vi "projectile_motion_MathScript_ver0.vi"() -> ()   [LabVIEW 2011]
uses:
  <vilib>/imath/engines/lvmath/Plug In/_Char/NIMS_CH_character datatype.ctl
  Instance           1 43Saved   Worked Example--Function Generation .vi
  <vilib>/Utility/file.llb/Write To Spreadsheet File (DBL).vi
  <vilib>/imath/engines/lvmath2/RunTimeEngine/ErrorHandling/NIMS_Finalize Error.vi
  <vilib>/imath/engines/lvmath2/RunTimeEngine/Managers/WorkSpace/UID Generator.vi
  <vilib>/imath/engines/lvmath2/RunTimeEngine/CommandStatement/NIMS_CommandStatement_MaskErr.vi
  <vilib>/imath/engines/lvmath2/RunTimeEngine/Managers/SymbolTable/Clear UID.vi
  <vilib>/imath/engines/lvmath2/RunTimeEngine/NodeEndStatement/NIMS_NodeEndStatement_Output.vi
  <instcachedir>/0/NIMS_NodeEndStatement_Output_53EC0D466D134D7ABD903AC30B43404B.lvgen/NIMS_NodeEndStatement_Output_53EC0D466D134D7ABD903AC30B43404B_001.vi
  <instcachedir>/0/NIMS_NodeEndStatement_Output_53EC0D466D134D7ABD903AC30B43404B.lvgen/NIMS_NodeEndStatement_Output_53EC0D466D134D7ABD903AC30B43404B_005.vi
  <vilib>/imath/engines/lvmath2/RunTimeEngine/ReplaceToken/NIMS_Replace - Check Linear.vi
  <instcachedir>/0/NIMS_Replace - Check Linear_276AD648BD064726893CCF9ED6E2A728.lvgen/NIMS_Replace - Check Linear_276AD648BD064726893CCF9ED6E2A728_006.vi
  <vilib>/imath/engines/lvmath2/RunTimeEngine/ReplaceToken/NIMS_Replace - Size Check _(_)=S.vi
  <instcachedir>/0/NIMS_Replace - Size Check _(_)=S_9ABE7AF2D26C43EAA05192D5C1E6C624.lvgen/NIMS_Replace - Size Check _(_)=S_9ABE7AF2D26C43EAA05192D5C1E6C624_004.vi
  <vilib>/imath/engines/lvmath2/RunTimeEngine/ReplaceToken/NIMS_Replace - V(S)=S.vi
  <instcachedir>/0/NIMS_Replace - V(S)=S_16B13A4565AB46F59881314645612498.lvgen/NIMS_Replace - V(S)=S_16B13A4565AB46F59881314645612498_002.vi
  <vilib>/imathl/engines/lvmath/Functions/Error Handling/Create Error.vi
  <instcachedir>/0/NIMS_Replace - Check Linear_276AD648BD064726893CCF9ED6E2A728.lvgen/NIMS_Replace - Check Linear_276AD648BD064726893CCF9ED6E2A728_001.vi
  <instcachedir>/0/NIMS_Replace - Size Check _(_)=S_9ABE7AF2D26C43EAA05192D5C1E6C624.lvgen/NIMS_Replace - Size Check _(_)=S_9ABE7AF2D26C43EAA05192D5C1E6C624_000.vi
  <instcachedir>/0/NIMS_Replace - V(S)=S_16B13A4565AB46F59881314645612498.lvgen/NIMS_Replace - V(S)=S_16B13A4565AB46F59881314645612498_000.vi
  <vilib>/imath/engines/lvmath2/RunTimeEngine/VariableToken/Read/NIMS_Get Elements - RV(_) - Check.vi
  <instcachedir>/0/NIMS_Get Elements - RV(_) - Check_B511B9D8E05044FE80F9F088FE24B20C.lvgen/NIMS_Get Elements - RV(_) - Check_B511B9D8E05044FE80F9F088FE24B20C_003.vi
  <vilib>/imath/engines/lvmath2/RunTimeEngine/CommandStatement/MC_CommandStatement_break.vi
  <instcachedir>/0/NIMS_Replace - Check Linear_276AD648BD064726893CCF9ED6E2A728.lvgen/NIMS_Replace - Check Linear_276AD648BD064726893CCF9ED6E2A728_002.vi
  <vilib>/imath/engines/lvmath2/RunTimeEngine/ArithmeticOperatorToken/NIMS_ArithmeticOperator_power(S).vi
  <instcachedir>/0/NIMS_ArithmeticOperator_power(S)_92C23AD9D71943099E05992575E16482.lvgen/NIMS_ArithmeticOperator_power(S)_92C23AD9D71943099E05992575E16482_010.vi
  <instcachedir>/0/NIMS_Replace - Size Check _(_)=S_9ABE7AF2D26C43EAA05192D5C1E6C624.lvgen/NIMS_Replace - Size Check _(_)=S_9ABE7AF2D26C43EAA05192D5C1E6C624_001.vi
  <instcachedir>/0/NIMS_Replace - V(S)=S_16B13A4565AB46F59881314645612498.lvgen/NIMS_Replace - V(S)=S_16B13A4565AB46F59881314645612498_001.vi
  <vilib>/imath/engines/lvmath2/RunTimeEngine/ErrorHandling/NIMS_Create Error From Enums.vi
  <instcachedir>/0/NIMS_Get Elements - RV(_) - Check_B511B9D8E05044FE80F9F088FE24B20C.lvgen/NIMS_Get Elements - RV(_) - Check_B511B9D8E05044FE80F9F088FE24B20C_000.vi
  <vilib>/imath/engines/lvmath2/RunTimeSupport/NIMS_Complex To Real.vi
  <instcachedir>/0/NIMS_Complex To Real_C6C689ECDA084B0290AC275552CC3682.lvgen/NIMS_Complex To Real_C6C689ECDA084B0290AC275552CC3682_003.vi
  <vilib>/imath/engines/lvmath2/RunTimeEngine/BuiltInFunctions/figure/NIMS_figure(I32).vi
  <vilib>/imath/engines/lvmath2/RunTimeEngine/BuiltInFunctions/plot/NIMS_plot(RM, RM, Str).vi
  <vilib>/imath/engines/lvmath2/RunTimeEngine/BuiltInFunctions/grid/NIMS_grid(Enums).vi
  <vilib>/imath/engines/lvmath/Plug In/_Char/NIMS_CH_Character RV to String.vi
  <vilib>/imath/engines/lvmath2/RunTimeEngine/BuiltInFunctions/title/NIMS_title.vi
  <vilib>/imath/engines/lvmath2/RunTimeEngine/BuiltInFunctions/xlabel/NIMS_xlabel.vi
  <vilib>/imath/engines/lvmath2/RunTimeEngine/BuiltInFunctions/ylabel/NIMS_ylabel.vi
  <vilib>/imath/engines/lvmath2/RunTimeEngine/BuiltInFunctions/plot/NIMS_plot(nRM, nRM).vi
  <vilib>/imath/engines/lvmath2/RunTimeEngine/BuiltInFunctions/legend/NIMS_legend(Arb).vi
  <vilib>/imath/engines/lvmath2/RunTimeEngine/Managers/SymbolTable/NIMS_WorkSpace.lvlib
panel:
  in  "delta_t":dbl[](array[numeric])=[0.5, 0.1, 0.01]
  out "Waveform Graph":cluster{dbl, "delta_t":dbl, dbl[][]}(graph)
  in  "Cd*C/m  (unitless)":dbl=0.001731
  in  "position_y0":dbl
  in  "position_x0":dbl
  out "XY Graph":cluster{"Y":dbl[], "Y":dbl[]}[](graph)=[{"Y"=[0.0, 63.65286717815624, 119.20727554453643, 168.9411686946953, 214.23953010967568, 255.97069455703536, 294.6722967050739, 330.6609696844568, 364.11046082675387, 0.0, 0.0, 0.0, 0.0, 0.0, 0.0, 0.0, 0.0, 0.0, 0.0, 0.0, 0.0, 0.0, 0.0, 0.0, 0.0, 0.0, 0.0, 0.0, 0.0, 0.0, 0.0, 0.0, 0.0, 0.0, 0.0, 0.0, 0.0, 0.0, 0.0, 0.0, 0.0, 0.0, 0.0, 0.0, 0.0, 0.0, 0.0, 0.0, 0.0, 0.0, 0.0, 0.0, 0.0, 0.0, 0.0, 0.0, 0.0, 0.0, 0.0, 0.0, 0.0, 0.0, 0.0, 0.0, 0.0, 0.0, 0.0, 0.0, 0.0, 0.0, 0.0, 0.0, 0.0, 0.0, 0.0, 0.0, 0.0, 0.0, 0.0, 0.0, 0.0, 0.0, 0.0, 0.0, 0.0, 0.0, 0.0, 0.0, 0.0, 0.0, 0.0, 0.0, 0.0, 0.0, 0.0, 0.0, 0.0, 0.0, 0.0, 0.0, 0.0, 0.0, 0.0, 0.0, 0.0, 0.0, 0.0, 0.0, 0.0, 0.0, 0.0, 0.0, 0.0, 0.0, 0.0, 0.0, 0.0, 0.0, 0.0, 0.0, 0.0, 0.0, 0.0, 0.0, 0.0, 0.0, 0.0, 0.0, 0.0, 0.0, 0.0, 0.0, 0.0, 0.0, 0.0, 0.0, 0.0, 0.0, 0.0, 0.0, 0.0, 0.0, 0.0, 0.0, 0.0, 0.0, 0.0, 0.0, 0.0, 0.0, 0.0, 0.0, 0.0, 0.0, 0.0, 0.0, 0.0, 0.0, 0.0, 0.0, 0.0, 0.0, 0.0, 0.0, 0.0, 0.0, 0.0, 0.0, 0.0, 0.0, 0.0, 0.0, 0.0, 0.0, 0.0, 0.0, 0.0, 0.0, 0.0, 0.0, 0.0, 0.0, 0.0, 0.0, 0.0, 0.0, 0.0, 0.0, 0.0, 0.0, 0.0, 0.0, 0.0, 0.0, 0.0, 0.0, 0.0, 0.0, 0.0, 0.0, 0.0, 0.0, 0.0, 0.0, 0.0, 0.0, 0.0, 0.0, 0.0, 0.0, 0.0, 0.0, 0.0, 0.0, 0.0, 0.0, 0.0, 0.0, 0.0, 0.0, 0.0, 0.0, 0.0, 0.0, 0.0, 0.0, 0.0, 0.0, 0.0, 0.0, 0.0, 0.0, 0.0, 0.0, 0.0, 0.0, 0.0, 0.0, 0.0, 0.0, 0.0, 0.0, 0.0, 0.0, 0.0, 0.0, 0.0, 0.0, 0.0, 0.0, 0.0, 0.0, 0.0, 0.0, 0.0, 0.0, 0.0, 0.0, 0.0, 0.0, 0.0, 0.0, 0.0, 0.0, 0.0, 0.0, 0.0, 0.0, 0.0, 0.0, 0.0, 0.0, 0.0, 0.0, 0.0, 0.0, 0.0, 0.0, 0.0, 0.0, 0.0, 0.0, 0.0, 0.0, 0.0, 0.0, 0.0, 0.0, 0.0, 0.0, 0.0, 0.0, 0.0, 0.0, 0.0, 0.0, 0.0, 0.0, 0.0, 0.0, 0.0, 0.0, 0.0, 0.0, 0.0, 0.0, 0.0, 0.0, 0.0, 0.0, 0.0, 0.0, 0.0, 0.0, 0.0, 0.0, 0.0, 0.0, 0.0, 0.0, 0.0, 0.0, 0.0, 0.0, 0.0, 0.0, 0.0, 0.0, 0.0, 0.0, 0.0, 0.0, 0.0, 0.0, 0.0, 0.0, 0.0, 0.0, 0.0, 0.0, 0.0, 0.0, 0.0, 0.0, 0.0, 0.0, 0.0, 0.0, 0.0, 0.0, 0.0, 0.0, 0.0, 0.0, 0.0, 0.0, 0.0, 0.0, 0.0, 0.0, 0.0, 0.0, 0.0, 0.0, 0.0, 0.0, 0.0, 0.0, 0.0, 0.0, 0.0, 0.0, 0.0, 0.0, 0.0, 0.0, 0.0, 0.0, 0.0, 0.0, 0.0, 0.0, 0.0, 0.0, 0.0, 0.0, 0.0, 0.0, 0.0, 0.0, 0.0, 0.0, 0.0, 0.0, 0.0, 0.0], "Y"=[0.0, 36.74999999999999, 60.774352624999985, 74.23163929383902, 78.438733934501, 74.26452442252095, 62.343350494005485, 43.20783448868342, 17.372425354815427, 0.0, 0.0, 0.0, 0.0, 0.0, 0.0, 0.0, 0.0, 0.0, 0.0, 0.0, 0.0, 0.0, 0.0, 0.0, 0.0, 0.0, 0.0, 0.0, 0.0, 0.0, 0.0, 0.0, 0.0, 0.0, 0.0, 0.0, 0.0, 0.0, 0.0, 0.0, 0.0, 0.0, 0.0, 0.0, 0.0, 0.0, 0.0, 0.0, 0.0, 0.0, 0.0, 0.0, 0.0, 0.0, 0.0, 0.0, 0.0, 0.0, 0.0, 0.0, 0.0, 0.0, 0.0, 0.0, 0.0, 0.0, 0.0, 0.0, 0.0, 0.0, 0.0, 0.0, 0.0, 0.0, 0.0, 0.0, 0.0, 0.0, 0.0, 0.0, 0.0, 0.0, 0.0, 0.0, 0.0, 0.0, 0.0, 0.0, 0.0, 0.0, 0.0, 0.0, 0.0, 0.0, 0.0, 0.0, 0.0, 0.0, 0.0, 0.0, 0.0, 0.0, 0.0, 0.0, 0.0, 0.0, 0.0, 0.0, 0.0, 0.0, 0.0, 0.0, 0.0, 0.0, 0.0, 0.0, 0.0, 0.0, 0.0, 0.0, 0.0, 0.0, 0.0, 0.0, 0.0, 0.0, 0.0, 0.0, 0.0, 0.0, 0.0, 0.0, 0.0, 0.0, 0.0, 0.0, 0.0, 0.0, 0.0, 0.0, 0.0, 0.0, 0.0, 0.0, 0.0, 0.0, 0.0, 0.0, 0.0, 0.0, 0.0, 0.0, 0.0, 0.0, 0.0, 0.0, 0.0, 0.0, 0.0, 0.0, 0.0, 0.0, 0.0, 0.0, 0.0, 0.0, 0.0, 0.0, 0.0, 0.0, 0.0, 0.0, 0.0, 0.0, 0.0, 0.0, 0.0, 0.0, 0.0, 0.0, 0.0, 0.0, 0.0, 0.0, 0.0, 0.0, 0.0, 0.0, 0.0, 0.0, 0.0, 0.0, 0.0, 0.0, 0.0, 0.0, 0.0, 0.0, 0.0, 0.0, 0.0, 0.0, 0.0, 0.0, 0.0, 0.0, 0.0, 0.0, 0.0, 0.0, 0.0, 0.0, 0.0, 0.0, 0.0, 0.0, 0.0, 0.0, 0.0, 0.0, 0.0, 0.0, 0.0, 0.0, 0.0, 0.0, 0.0, 0.0, 0.0, 0.0, 0.0, 0.0, 0.0, 0.0, 0.0, 0.0, 0.0, 0.0, 0.0, 0.0, 0.0, 0.0, 0.0, 0.0, 0.0, 0.0, 0.0, 0.0, 0.0, 0.0, 0.0, 0.0, 0.0, 0.0, 0.0, 0.0, 0.0, 0.0, 0.0, 0.0, 0.0, 0.0, 0.0, 0.0, 0.0, 0.0, 0.0, 0.0, 0.0, 0.0, 0.0, 0.0, 0.0, 0.0, 0.0, 0.0, 0.0, 0.0, 0.0, 0.0, 0.0, 0.0, 0.0, 0.0, 0.0, 0.0, 0.0, 0.0, 0.0, 0.0, 0.0, 0.0, 0.0, 0.0, 0.0, 0.0, 0.0, 0.0, 0.0, 0.0, 0.0, 0.0, 0.0, 0.0, 0.0, 0.0, 0.0, 0.0, 0.0, 0.0, 0.0, 0.0, 0.0, 0.0, 0.0, 0.0, 0.0, 0.0, 0.0, 0.0, 0.0, 0.0, 0.0, 0.0, 0.0, 0.0, 0.0, 0.0, 0.0, 0.0, 0.0, 0.0, 0.0, 0.0, 0.0, 0.0, 0.0, 0.0, 0.0, 0.0, 0.0, 0.0, 0.0, 0.0, 0.0, 0.0, 0.0, 0.0, 0.0, 0.0, 0.0, 0.0, 0.0, 0.0, 0.0, 0.0, 0.0, 0.0, 0.0, 0.0, 0.0, 0.0, 0.0, 0.0, 0.0, 0.0, 0.0, 0.0, 0.0, 0.0, 0.0, 0.0, 0.0, 0.0, 0.0, 0.0, 0.0, 0.0, 0.0, 0.0, 0.0, 0.0, 0.0, 0.0, 0.0, 0.0, 0.0, 0.0, 0.0, 0.0, 0.0, 0.0, 0.0, 0.0, 0.0, 0.0]}, {"Y"=[0.0, 12.73057343563125, 25.137208518791457, 37.23957985485345, 49.055624386148914, 60.60172756357031, 71.89288391369205, 82.9428360767805, 93.76419566069593, 104.36854867446878, 114.76654784008252, 124.96799370649973, 134.98190618687568, 144.81658789322674, 154.47968044082782, 163.97821472803884, 173.31865605871113, 182.50694485786246, 191.548533632143, 200.4484207408846, 209.21118146815996, 217.8409968188849, 226.341680400791, 234.7167036978456, 242.96921998864292, 251.10208711510637, 259.11788926251256, 267.01895787160345, 274.80739176773767, 282.48507656101253, 290.05370334535553, 297.5147867038768, 304.86968201224676, 312.11960202126164, 319.26563269364624, 326.30874826793575, 333.2498255232935, 340.0896572226416, 346.8289647167974, 353.4684096987675, 360.0086051043837, 0.0, 0.0, 0.0, 0.0, 0.0, 0.0, 0.0, 0.0, 0.0, 0.0, 0.0, 0.0, 0.0, 0.0, 0.0, 0.0, 0.0, 0.0, 0.0, 0.0, 0.0, 0.0, 0.0, 0.0, 0.0, 0.0, 0.0, 0.0, 0.0, 0.0, 0.0, 0.0, 0.0, 0.0, 0.0, 0.0, 0.0, 0.0, 0.0, 0.0, 0.0, 0.0, 0.0, 0.0, 0.0, 0.0, 0.0, 0.0, 0.0, 0.0, 0.0, 0.0, 0.0, 0.0, 0.0, 0.0, 0.0, 0.0, 0.0, 0.0, 0.0, 0.0, 0.0, 0.0, 0.0, 0.0, 0.0, 0.0, 0.0, 0.0, 0.0, 0.0, 0.0, 0.0, 0.0, 0.0, 0.0, 0.0, 0.0, 0.0, 0.0, 0.0, 0.0, 0.0, 0.0, 0.0, 0.0, 0.0, 0.0, 0.0, 0.0, 0.0, 0.0, 0.0, 0.0, 0.0, 0.0, 0.0, 0.0, 0.0, 0.0, 0.0, 0.0, 0.0, 0.0, 0.0, 0.0, 0.0, 0.0, 0.0, 0.0, 0.0, 0.0, 0.0, 0.0, 0.0, 0.0, 0.0, 0.0, 0.0, 0.0, 0.0, 0.0, 0.0, 0.0, 0.0, 0.0, 0.0, 0.0, 0.0, 0.0, 0.0, 0.0, 0.0, 0.0, 0.0, 0.0, 0.0, 0.0, 0.0, 0.0, 0.0, 0.0, 0.0, 0.0, 0.0, 0.0, 0.0, 0.0, 0.0, 0.0, 0.0, 0.0, 0.0, 0.0, 0.0, 0.0, 0.0, 0.0, 0.0, 0.0, 0.0, 0.0, 0.0, 0.0, 0.0, 0.0, 0.0, 0.0, 0.0, 0.0, 0.0, 0.0, 0.0, 0.0, 0.0, 0.0, 0.0, 0.0, 0.0, 0.0, 0.0, 0.0, 0.0, 0.0, 0.0, 0.0, 0.0, 0.0, 0.0, 0.0, 0.0, 0.0, 0.0, 0.0, 0.0, 0.0, 0.0, 0.0, 0.0, 0.0, 0.0, 0.0, 0.0, 0.0, 0.0, 0.0, 0.0, 0.0, 0.0, 0.0, 0.0, 0.0, 0.0, 0.0, 0.0, 0.0, 0.0, 0.0, 0.0, 0.0, 0.0, 0.0, 0.0, 0.0, 0.0, 0.0, 0.0, 0.0, 0.0, 0.0, 0.0, 0.0, 0.0, 0.0, 0.0, 0.0, 0.0, 0.0, 0.0, 0.0, 0.0, 0.0, 0.0, 0.0, 0.0, 0.0, 0.0, 0.0, 0.0, 0.0, 0.0, 0.0, 0.0, 0.0, 0.0, 0.0, 0.0, 0.0, 0.0, 0.0, 0.0, 0.0, 0.0, 0.0, 0.0, 0.0, 0.0, 0.0, 0.0, 0.0, 0.0, 0.0, 0.0, 0.0, 0.0, 0.0, 0.0, 0.0, 0.0, 0.0, 0.0, 0.0, 0.0, 0.0, 0.0, 0.0, 0.0, 0.0, 0.0, 0.0, 0.0, 0.0, 0.0, 0.0, 0.0, 0.0, 0.0, 0.0, 0.0, 0.0, 0.0, 0.0, 0.0, 0.0, 0.0, 0.0, 0.0, 0.0, 0.0, 0.0, 0.0, 0.0, 0.0, 0.0, 0.0, 0.0, 0.0, 0.0, 0.0, 0.0, 0.0, 0.0, 0.0, 0.0, 0.0, 0.0, 0.0, 0.0, 0.0, 0.0, 0.0, 0.0, 0.0, 0.0, 0.0, 0.0, 0.0, 0.0, 0.0, 0.0, 0.0, 0.0, 0.0, 0.0, 0.0, 0.0, 0.0, 0.0, 0.0, 0.0, 0.0, 0.0, 0.0, 0.0], "Y"=[0.0, 7.349999999999999, 14.190974104999997, 20.542178270686286, 26.421120975648577, 31.84375733563033, 36.82465771938414, 41.377155004066154, 45.513473863301236, 49.24484488574205, 52.58160584244948, 55.53329203215366, 58.10871731483205, 60.31604718098245, 62.162864984808365, 63.656232285230956, 64.80274408220603, 65.60857960188835, 66.07954916868616, 66.2211376021788, 66.03854449007372, 65.5367216133773, 64.72040773578085, 63.59416091530972, 62.16238845214948, 60.42937455191681, 58.39930575810012, 56.07629419042934, 53.46439861681772, 50.56764338430642, 47.390035237997125, 43.93557806500312, 40.208285611648975, 36.2121922351912, 31.95136176501055, 27.429894561503215, 22.65193287294656, 17.621664600837235, 12.34332559222224, 6.821200583194698, 1.0596229210023012, 0.0, 0.0, 0.0, 0.0, 0.0, 0.0, 0.0, 0.0, 0.0, 0.0, 0.0, 0.0, 0.0, 0.0, 0.0, 0.0, 0.0, 0.0, 0.0, 0.0, 0.0, 0.0, 0.0, 0.0, 0.0, 0.0, 0.0, 0.0, 0.0, 0.0, 0.0, 0.0, 0.0, 0.0, 0.0, 0.0, 0.0, 0.0, 0.0, 0.0, 0.0, 0.0, 0.0, 0.0, 0.0, 0.0, 0.0, 0.0, 0.0, 0.0, 0.0, 0.0, 0.0, 0.0, 0.0, 0.0, 0.0, 0.0, 0.0, 0.0, 0.0, 0.0, 0.0, 0.0, 0.0, 0.0, 0.0, 0.0, 0.0, 0.0, 0.0, 0.0, 0.0, 0.0, 0.0, 0.0, 0.0, 0.0, 0.0, 0.0, 0.0, 0.0, 0.0, 0.0, 0.0, 0.0, 0.0, 0.0, 0.0, 0.0, 0.0, 0.0, 0.0, 0.0, 0.0, 0.0, 0.0, 0.0, 0.0, 0.0, 0.0, 0.0, 0.0, 0.0, 0.0, 0.0, 0.0, 0.0, 0.0, 0.0, 0.0, 0.0, 0.0, 0.0, 0.0, 0.0, 0.0, 0.0, 0.0, 0.0, 0.0, 0.0, 0.0, 0.0, 0.0, 0.0, 0.0, 0.0, 0.0, 0.0, 0.0, 0.0, 0.0, 0.0, 0.0, 0.0, 0.0, 0.0, 0.0, 0.0, 0.0, 0.0, 0.0, 0.0, 0.0, 0.0, 0.0, 0.0, 0.0, 0.0, 0.0, 0.0, 0.0, 0.0, 0.0, 0.0, 0.0, 0.0, 0.0, 0.0, 0.0, 0.0, 0.0, 0.0, 0.0, 0.0, 0.0, 0.0, 0.0, 0.0, 0.0, 0.0, 0.0, 0.0, 0.0, 0.0, 0.0, 0.0, 0.0, 0.0, 0.0, 0.0, 0.0, 0.0, 0.0, 0.0, 0.0, 0.0, 0.0, 0.0, 0.0, 0.0, 0.0, 0.0, 0.0, 0.0, 0.0, 0.0, 0.0, 0.0, 0.0, 0.0, 0.0, 0.0, 0.0, 0.0, 0.0, 0.0, 0.0, 0.0, 0.0, 0.0, 0.0, 0.0, 0.0, 0.0, 0.0, 0.0, 0.0, 0.0, 0.0, 0.0, 0.0, 0.0, 0.0, 0.0, 0.0, 0.0, 0.0, 0.0, 0.0, 0.0, 0.0, 0.0, 0.0, 0.0, 0.0, 0.0, 0.0, 0.0, 0.0, 0.0, 0.0, 0.0, 0.0, 0.0, 0.0, 0.0, 0.0, 0.0, 0.0, 0.0, 0.0, 0.0, 0.0, 0.0, 0.0, 0.0, 0.0, 0.0, 0.0, 0.0, 0.0, 0.0, 0.0, 0.0, 0.0, 0.0, 0.0, 0.0, 0.0, 0.0, 0.0, 0.0, 0.0, 0.0, 0.0, 0.0, 0.0, 0.0, 0.0, 0.0, 0.0, 0.0, 0.0, 0.0, 0.0, 0.0, 0.0, 0.0, 0.0, 0.0, 0.0, 0.0, 0.0, 0.0, 0.0, 0.0, 0.0, 0.0, 0.0, 0.0, 0.0, 0.0, 0.0, 0.0, 0.0, 0.0, 0.0, 0.0, 0.0, 0.0, 0.0, 0.0, 0.0, 0.0, 0.0, 0.0, 0.0, 0.0, 0.0, 0.0, 0.0, 0.0, 0.0, 0.0, 0.0, 0.0, 0.0, 0.0, 0.0, 0.0, 0.0, 0.0, 0.0, 0.0, 0.0, 0.0, 0.0, 0.0, 0.0, 0.0, 0.0, 0.0, 0.0, 0.0, 0.0, 0.0, 0.0, 0.0, 0.0, 0.0, 0.0, 0.0, 0.0]}, {"Y"=[0.0, 1.273057343563125, 2.5428753036015395, 3.8094738778503183, 5.072872882311105, 6.333091953312255, 7.59015054953858, 8.844067954031235, 10.09486327615826, 11.342555453556283, 12.587163254043872, 13.828705277507064, 15.067199957757483, 16.30266556436358, 17.535120204455414, 18.764581824503434, 19.991068212071717, 21.214596997546064, 22.435185655837415, 23.652851508060976, 24.867611723191466, 26.07948331969488, 27.288483167137194, 28.494627987770347, 29.69793435809591, 30.8984187104068, 32.096097334307416, 33.29098637821252, 34.483101850825264, 35.67245962259464, 36.859075427152746, 38.04296486273219, 39.22414339356391, 40.40262635125578, 41.57842893615231, 42.75156621867566, 43.92205314064846, 45.08990451659846, 46.25513503504558, 47.41775925977145, 48.577791631071754, 49.73524646699175, 50.8901379645451, 52.042480200916394, 53.192287134647515, 54.33957260680819, 55.48435034215093, 56.62663395025064, 57.76643692662907, 58.903772653864436, 60.03865440268638, 61.17109533305652, 62.3011084952348, 63.4287068308319, 64.55390317384786, 65.67671025169717, 66.79714068622059, 67.91520699468373, 69.03092159076284, 70.1442967855178, 71.25534478835257, 72.36407770796338, 73.47050755327467, 74.57464623436321, 75.6765055633703, 76.77609725540242, 77.87343292942053, 78.96852410911802, 80.06138222378763, 81.15201860917746, 82.24044450833621, 83.3266710724479, 84.41070936165606, 85.4925703458778, 86.57226490560758, 87.64980383271121, 88.72519783120993, 89.79845751805482, 90.86959342389177, 91.93861599381701, 93.00553558812341, 94.07036248303771, 95.13310687144879, 96.19377886362703, 97.25238848793512, 98.30894569153018, 99.36346034105746, 100.4159422233358, 101.46640104603482, 102.51484643834404, 103.56128795163414, 104.6057350601103, 105.64819716145786, 106.68868357748033, 107.72720355473005, 108.76376626513128, 109.7983808065962, 110.83105620363362, 111.86180140795074, 112.89062529904785, 113.91753668480635, 114.94254430206979, 115.96565681721849, 116.9868828267375, 118.00623085777812, 119.0237093687131, 120.03932674968556, 121.05309132315173, 122.06501134441767, 123.0750950021699, 124.0833504190003, 125.08978565192501, 126.09440869289782, 127.09722746931769, 128.09824984453093, 129.09748361832777, 130.09493652743367, 131.0906162459952, 132.0845303860607, 133.07668649805595, 134.06709207125456, 135.05575453424356, 136.04268125538385, 137.02787954326604, 138.01135664716134, 138.99311975746787, 139.97317600615227, 140.95153246718675, 141.9281961569817, 142.90317403481384, 143.87647300325003, 144.8480999085668, 145.8180615411657, 146.78636463598428, 147.75301587290335, 148.71802187714988, 149.68138921969606, 150.6431244176545, 151.60323393466945, 152.5617241813044, 153.51860151542587, 154.4738722425834, 155.42754261638626, 156.37961883887618, 157.330107060897, 158.27901338246056, 159.2263438531093, 160.17210447227566, 161.11630118963797, 162.0589399054732, 163.00002647100663, 163.93956668875825, 164.87756631288613, 165.81403104952676, 166.74896655713243, 167.68237844680567, 168.61427228263074, 169.54465358200235, 170.47352781595163, 171.40090040946916, 172.32677674182554, 173.25116214688916, 174.17406191344136, 175.09548128548903, 176.0154254625747, 176.9338996000842, 177.85090880955167, 178.76645815896237, 179.68055267305309, 180.59319733361014, 181.50439707976508, 182.41415680828834, 183.32248137388035, 184.2293755894608, 185.13484422645556, 186.03889201508153, 186.9415236446295, 187.84274376374498, 188.7425569807068, 189.64096786370416, 190.53798094111139, 191.4336007017609, 192.32783159521443, 193.22067803203234, 194.11214438404096, 195.00223498459846, 195.8909541288588, 196.778306074034, 197.66429503965472, 198.54892520782923, 199.43220072350067, 200.3141256947029, 201.19470419281453, 202.07394025281155, 202.95183787351854, 203.82840101785817, 204.70363361309936, 205.57753955110402, 206.45012268857238, 207.3213868472868, 208.19133581435435, 209.05997334244807, 209.9273031500468, 210.79332892167378, 211.6580543081338, 212.52148292674954, 213.38361836159612, 214.24446416373485, 215.10402385144556, 215.96230091045788, 216.81929879418135, 217.67502092393428, 218.52947068917166, 219.3826514477118, 220.23456652596207, 221.08521921914343, 221.93461279151398, 222.7827504765915, 223.62963547737482, 224.47527096656444, 225.319660086782, 226.16280595078877, 227.00471164170324, 227.8453802132178, 228.6848146898144, 229.52301806697935, 230.35999331141724, 231.1957433612639, 232.03027112629857, 232.86357948815507, 233.6956713005323, 234.52654938940373, 235.35621655322618, 236.18467556314764, 237.01192916321443, 237.8379800705775, 238.6628309756978, 239.48648454255115, 240.30894340883205, 241.13021018615686, 241.95028746026625, 242.76917779122684, 243.58688371363203, 244.40340773680225, 245.21875234498435, 246.03291999755032, 246.84591312919528, 247.6577341501348, 248.4683854463013, 249.27786937954025, 250.08618828780493, 250.89334448535124, 251.69934026293132, 252.50417788798669, 253.3078596048407, 254.11038763489032, 254.91176417679705, 255.71199140667756, 256.5110714782933, 257.3090065232395, 258.10579865113374, 258.9014499498038, 259.6959624854744, 260.489338302954, 261.2815794258205, 262.0726878566062, 262.8626655769825, 263.6515145479438, 264.4392367099905, 265.2258339833116, 266.0113082679667, 266.7956614440671, 267.5788953719566, 268.36101189239133, 269.14201282671905, 269.9218999770579, 270.7006751264743, 271.47834003916057, 272.25489646061135, 273.03034611779987, 273.80469071935323, 274.5779319557274, 275.3500714993811, 276.12111100494934, 276.89105210941625, 277.65989643228727, 278.42764557576055, 279.1943011248979, 279.95986464779475, 280.72433769574985, 281.4877218034341, 282.2500184890586, 283.01122925454223, 283.7713555856784, 284.53039895230125, 285.2883608084511, 286.0452425925393, 286.8010457275122, 287.5557716210147, 288.3094216655529, 289.0619972386562, 289.8134997030386, 290.56393040675925, 291.31329068338266, 292.06158185213764, 292.8088052180761, 293.5549620722307, 294.3000536917721, 295.04408134016535, 295.7870462673254, 296.52894970977235, 297.2697928907855, 298.00957702055695, 298.74830329634443, 299.48597290262325, 300.22258701123775, 300.9581467815518, 301.6926533605988, 302.4261078832306, 303.15851147226596, 303.8898652386382, 304.6201702815421, 305.34942768857974, 306.07763853590626, 306.8048038883741, 307.53092479967717, 308.2560023124935, 308.9800374586279, 309.7030312591535, 310.4249847245521, 311.1458988548546, 311.86577463977994, 312.58461305887374, 313.30241508164573, 314.01918166770673, 314.73491376690464, 315.44961231945985, 316.1632782560996, 316.8759124981917, 317.58751595787754, 318.29808953820407, 319.0076341332551, 319.716150628282, 320.42363989983306, 321.1301028158828, 321.8355402359597, 322.5399530112736, 323.2433419848423, 323.945707991617, 324.64705185860737, 325.34737440500544, 326.0466764423088, 326.74495877444315, 327.44222219788367, 328.13846750177606, 328.83369546805625, 329.5279068715696, 330.2211024801893, 330.9132830549337, 331.604449350083, 332.2946021132952, 332.983742085721, 333.67187000211817, 334.35898659096455, 335.0450925745709, 335.73018866919256, 336.4142755851402, 337.09735402689006, 337.779424693193, 338.4604882771831, 339.1405454664851, 339.8195969433211, 340.4976433846167, 341.17468546210597, 341.8507238424357, 342.5257591872689, 343.1997921533874, 343.8728233927938, 344.5448535528122, 345.21588327618855, 345.88591320118985, 346.55494396170286, 347.2229761873316, 347.89001050349435, 348.5560475315196, 349.2210878887414, 349.88513218859384, 350.54818104070443, 351.2102350509871, 351.87129482173407, 352.53136095170714, 353.19043403622805, 353.8485146672679, 354.50560343353607, 355.161700920568, 355.8168077108126], "Y"=[0.0, 0.7349999999999999, 1.4649097410499998, 2.1897489325551014, 2.9095370991203025, 3.6242935827044103, 4.334037544743263, 5.038787968242807, 5.7385636598425505, 6.433383251849932, 7.123265204246097, 7.808227806663599, 8.488289180336496, 9.163467280023351, 9.833779895903573, 10.499244655447598, 11.159879025261326, 11.815700312905296, 12.466725668688994, 13.112972087440758, 13.75445641025367, 14.39119532620787, 15.023205374069661, 15.650502943967853, 16.273104279047665, 16.891025477102623, 17.504282492184803, 18.112891136193777, 18.71686708044463, 19.316225857215397, 19.910982861274288, 20.50115335138698, 21.086752451804372, 21.66779515373111, 22.244296316775152, 22.81627067037879, 23.383732815231323, 23.94669722466377, 24.50517824602587, 25.059190102045687, 25.60874689217208, 26.153862593900346, 26.694551064081313, 27.230826040214108, 27.762701141722907, 28.290189871217947, 28.813305615740983, 29.33206164799552, 29.846471127562012, 30.356547102098293, 30.86230250852549, 31.363750174199623, 31.86090281806912, 32.35377305181854, 32.842373380998616, 33.32671620614291, 33.806813823871316, 34.282678427980514, 34.754322110521706, 35.22175686286574, 35.6849945767559, 36.144047045348465, 36.59892596424133, 37.04964293249081, 37.49620945361683, 37.93863693659666, 38.37693669684747, 38.81111995719775, 39.24119784884781, 39.66718141231964, 40.0890815983961, 40.506909269049764, 40.92067519836153, 41.33039007342911, 41.73606449526562, 42.137708979688426, 42.53533395819829, 42.9289497788491, 43.31856670710829, 43.70419492670799, 44.08584454048723, 44.46352557122515, 44.8372479624655, 45.20702157933246, 45.572856209338006, 45.93476156318081, 46.292747275536975, 46.646822905842605, 46.99699793906836, 47.34328178648615, 47.685683786428065, 48.02421320503761, 48.358879237013475, 48.68969100634581, 49.01665756704526, 49.339787903864725, 49.659090933014085, 49.974575502867886, 50.286250394666176, 50.59412432320852, 50.89820593754135, 51.19850382163872, 51.49502649507655, 51.78778241370053, 52.07677997028764, 52.36202749520149, 52.643533257041575, 52.921305463286444, 53.19535226093093, 53.465681737117535, 53.73230191976201, 53.995220778173284, 54.25444622366773, 54.509986110177906, 54.761848234855876, 55.01004033867109, 55.254570107003005, 55.49544517022848, 55.732673104303956, 55.96626143134262, 56.19621762018653, 56.422549086973746, 56.645263195700664, 56.86436725877949, 57.07986853759095, 57.29177424303238, 57.50009153606115, 57.70482752823354, 57.90598928223911, 58.10358381243069, 58.29761808534991, 58.48809902024846, 58.67503348960512, 58.858428319638485, 59.038290290815624, 59.21462613835662, 59.38744255273503, 59.55674618017439, 59.72254362314076, 59.884841440831345, 60.04364614965934, 60.19896422373488, 60.350802095342345, 60.49916615541385, 60.64406275399916, 60.78549820073192, 60.92347876529239, 61.058010677866534, 61.189100129601734, 61.31675327305898, 61.44097622266166, 61.561775055141, 61.67915580997815, 61.79312448984298, 61.9036870610296, 62.01084945388868, 62.114617563256566, 62.21499724888122, 62.31199433584507, 62.40561461498476, 62.49586384330782, 62.58274774440633, 62.66627200886759, 62.74644229468177, 62.823264227646725, 62.8967434017698, 62.96688537966678, 63.03369569295802, 63.09717984266171, 63.15734329958433, 63.214191504708374, 63.26772986957724, 63.31796377667747, 63.36489857981826, 63.40853960450823, 63.448892148329605, 63.48596148130973, 63.51975284628994, 63.55027145929185, 63.57752250988108, 63.601511161528386, 63.62224255196827, 63.63972179355507, 63.65395397361651, 63.6649441548048, 63.67269737544524, 63.67721864988238, 63.67851296882372, 63.676585299681, 63.671440586909085, 63.66308375234242, 63.65151969552914, 63.636753294062764, 63.618789403911606, 63.59763285974576, 63.57328847526179, 63.54576104350512, 63.51505533719004, 63.48117610901754, 63.444128091990706, 63.40391599972795, 63.36054452677392, 63.31401834890817, 63.26434212345157, 63.211520489570475, 63.155558068578664, 63.096459464237064, 63.034229263051245, 62.968872034566694, 62.90039233166193, 62.82879469083935, 62.754083632514, 62.67626366130003, 62.59533926629505, 62.51131492136235, 62.42419508541086, 62.33398420267301, 62.24068670298044, 62.14430700203754, 62.04484950169285, 61.94231859020832, 61.83671864252644, 61.728054020535225, 61.61632907333111, 61.50154813747965, 61.38371553727419, 61.26283558499234, 61.138912581150365, 61.0119508147555, 60.88195456355609, 60.748928094289695, 60.61287566292902, 60.47380151492582, 60.331709885452646, 60.18660499964257, 60.038491072826716, 59.88737231076981, 59.73325290990357, 59.57613705755803, 59.416028932190805, 59.25293270361424, 59.08685253322051, 58.91779257420461, 58.74575697178532, 58.57074986342404, 58.39277537904161, 58.211837641233, 58.02794076547998, 57.841088860361744, 57.65128602776336, 57.45853636308232, 57.262843955432864, 57.064212887848406, 56.86264723748176, 56.65815107580341, 56.450728468797685, 56.24038347715689, 56.02712015647339, 55.81094255742965, 55.59185472598624, 55.36986070356777, 55.14496452724681, 54.91717022992579, 54.68648184051678, 54.45290338411935, 54.21643888219635, 53.97709235274761, 53.734867810481724, 53.489769266985704, 53.241800730892706, 52.990966208047666, 52.73726970167097, 52.48071521252009, 52.22130673904924, 51.95904827756699, 51.693943822391915, 51.42599736600622, 51.155212899207406, 50.88159441125791, 50.60514589003278, 50.325871322165376, 50.04377469319108, 49.75885998768905, 49.47113118942197, 49.18059228147388, 48.88724724638604, 48.591100066290814, 48.29215472304362, 47.99041519835297, 47.685885473908485, 47.378569531507075, 47.068471353177145, 46.75559492130087, 46.43994421873456, 46.121523228927146, 45.80033593603671, 45.47638632504517, 45.149678381871034, 44.82021609348028, 44.48800344799537, 44.15304443480236, 43.81534304465621, 43.47490326978415, 43.13172910398726, 42.78582454274019, 42.437193583289, 42.08584022474728, 41.73176846819031, 41.37498231674752, 41.01548577569307, 40.65328285253471, 40.28837755710074, 39.92077390162531, 39.55047590083187, 39.17748757201488, 38.80181293511978, 38.42345601282115, 38.04242083059924, 37.65871141681469, 37.272331802781544, 36.88328602283857, 36.491578114418886, 36.09721211811788, 35.700192077759446, 35.30052204046056, 34.898206056694185, 34.493248180350555, 34.085652468796766, 33.675422982934776, 33.262563787257776, 32.84707894990493, 32.42897254271456, 32.00824864127568, 31.584911324978002, 31.15896467706036, 30.730412784657567, 30.29925973884573, 29.865509634686035, 29.429166571266997, 28.990234651745215, 28.54871798338461, 28.104620677594173, 27.65794684996424, 27.208700620301293, 26.756886112661316, 26.302507455381686, 25.84556878111166, 25.386074226841398, 24.924027933929633, 24.459434048129882, 23.99229671961532, 23.522620103002254, 23.050408357372234, 22.575665646292833, 22.098396137837067, 21.618604004601497, 21.136293423723018, 20.651468576894352, 20.164133650378233, 19.67429283502033, 19.181950326260907, 18.687110324145202, 18.18977703333261, 17.689954663104594, 17.187647427371402, 16.68285954467758, 16.175595238206284, 15.665858735782423, 15.153654269874618, 14.638986077596027, 14.121858400704012, 13.602275485598685, 13.080241583320333, 12.555760949545734, 12.028837844583384, 11.49947653336765, 10.967681285451839, 10.433456375000224, 9.896806080779026, 9.357734686146353, 8.816246479041137, 8.27234575197105, 7.726036801999439, 7.177323930731262, 6.6262114442980735, 6.072703653342037, 5.516804872999004, 4.95851942288065, 4.3978516270556955, 3.8348058140302173, 3.2693863167270623, 2.7015974724643774, 2.131443622933266, 1.5589291141745838, 0.984058296554888, 0.40683552474154694]}]
  in  "angle from horizon\n(degrees)":dbl=30.0
  in  "Velocity_0\n(ft/sec)":dbl=147.0
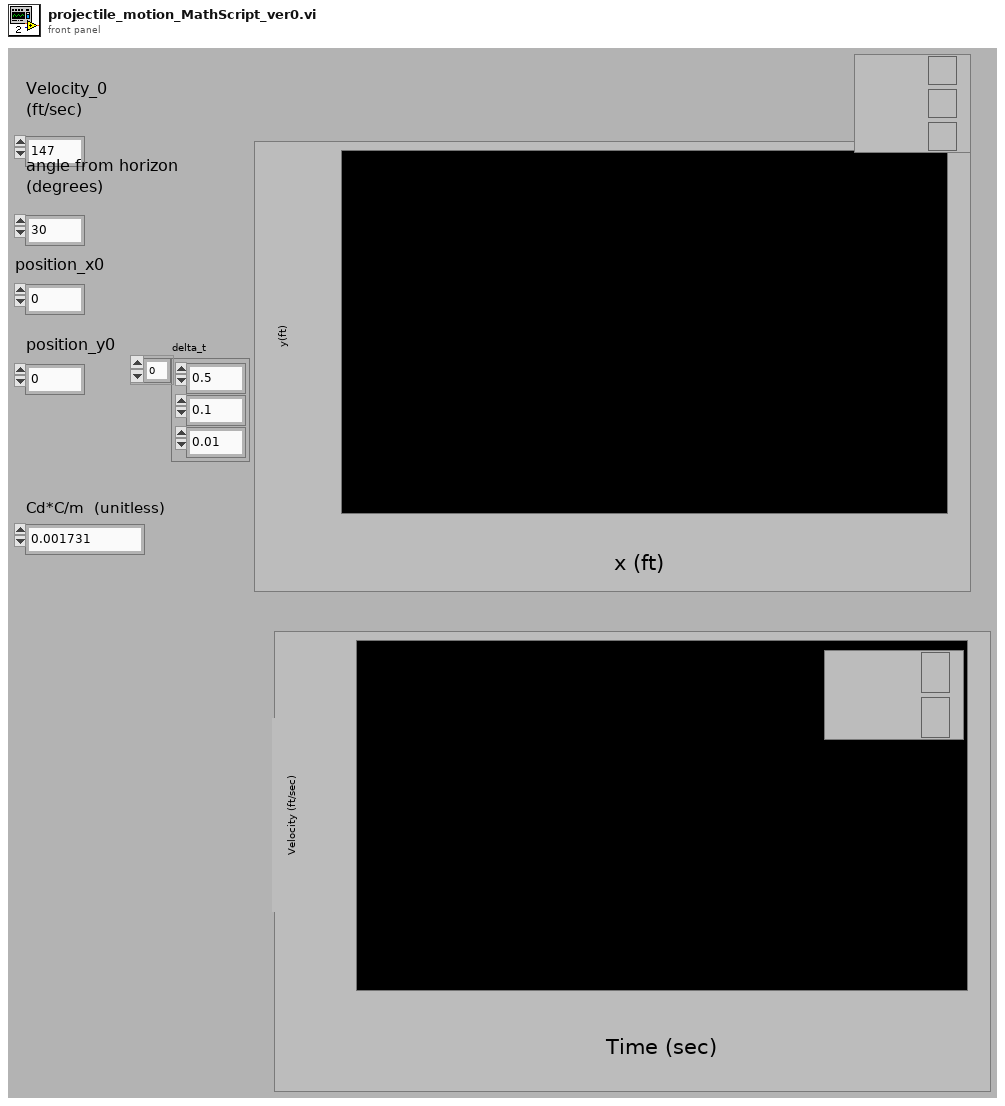
[diagram p1: front panel]
types:
  T1 = typedef "NIMS_CH_character datatype.ctl" = cluster{"Numeric":u8}
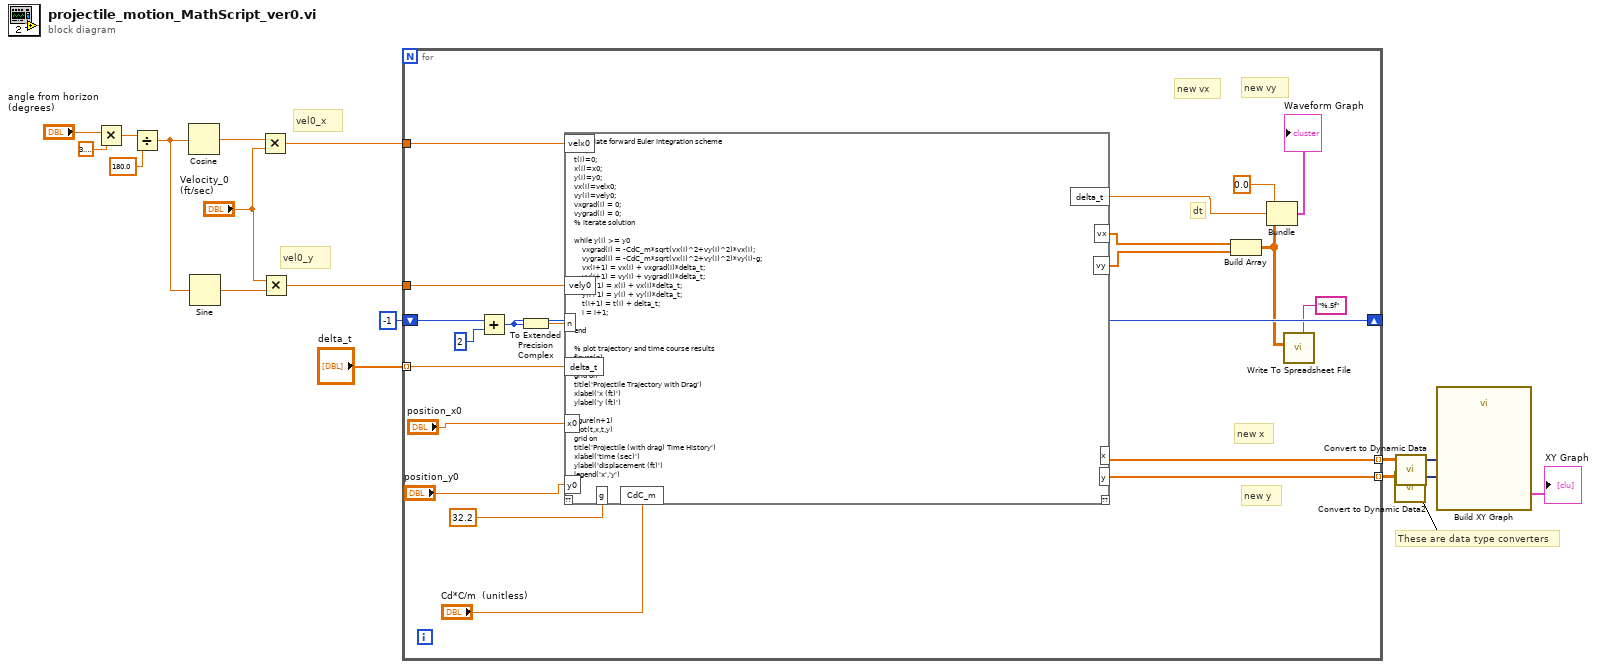
[diagram p0: block diagram]
diagram:
  # "vel0_y"
  # "vel0_x"
  # "These are data type converters"
  n1 = Multiply(x="angle from horizon\n(degrees)", y=3.141592653589793) -> (x*y=w12:dbl)
  n2 = Divide(x=w12, y=180.0) -> (x/y=w10:dbl)
  n3 = Cosine(x=w10) -> (cos(x)=w7:dbl)
  n4 = Sine(x=w10) -> (sin(x)=w9:dbl)
  n5 = Multiply(x=w7, y="Velocity_0\n(ft/sec)") -> (x*y=w5:dbl)
  n6 = Multiply(x="Velocity_0\n(ft/sec)", y=w9) -> (x*y=w6:dbl)
  n7 = for {
    tunnel: w6 -> [w32]
    tunnel: w5 -> [w31]
    tunnel: "delta_t" -> [w28] mode=indexing
    tunnel: [w30] -> w3 mode=indexing
    tunnel: [w29] -> w2 mode=indexing
    shift-right: [w20] -> _
    shift-left: -1 -> [w22]
    # "dt"
    # "new y"
    # "new x"
    # "new vy"
    # "new vx"
    n8 = Add(x=w22, y=2) -> (x+y=w20:i32)
    n9 = To Extended Precision Complex(1:w20) -> (0:w27:cxt)
    n10 = mathscript code="% initiate forward Euler integration scheme\ni=1;\nt(i)=0;\nx(i)=x0;\ny(i)=y0;\nvx(i)=velx0;\nvy(i)=vely0;\nvxgrad(i) = 0;\nvygrad(i) = 0;\n% iterate solution\n\nwhile y(i) >= y0    \n    vxgrad(i) = -CdC_m*sqrt(vx(i)^2+vy(i)^2)*vx(i);\n    vygrad(i) = -CdC_m*sqrt(vx(i)^2+vy(i)^2)*vy(i)-g;\n    vx(i+1) = vx(i) + vxgrad(i)*delta_t;\n    vy(i+1) = vy(i) + vygrad(i)*delta_t;\n    x(i+1) = x(i) + vx(i)*delta_t;\n    y(i+1) = y(i) + vy(i)*delta_t;\n    t(i+1) = t(i) + delta_t;\n    i = i+1;\n    \nend\n\n% plot trajectory and time course results\nfigure(n)\nplot(x,y)\ngrid on\ntitle('Projectile Trajectory with Drag')\nxlabel('x (ft)')\nylabel('y (ft)')\n\nfigure(n+1)\nplot(t,x,t,y)\ngrid on\ntitle('Projectile (with drag) Time History')\nxlabel('time (sec)')\nylabel('displacement (ft)')\nlegend('x','y')"("x0"="position_x0", "y0"="position_y0", "velx0"=w31, "vely0"=w32, "g"=32.2 ("y"), "CdC_m"="Cd*C/m  (unitless)", "delta_t"=w28, "n"=w27) -> ("vx"=w26:dbl[], "vy"=w25:dbl[], "x"=w30:dbl[], "y"=w29:dbl[], "delta_t"=w24:dbl)  [unwired: 1 in, 1 out]
    n11 = Build Array(w26, w25) -> (w18:dbl[][])
    n12 = Bundle(0.0, "delta_t"=w24, w18) -> (→"Waveform Graph":cluster{dbl, "delta_t":dbl, dbl[][]})  [unwired: 1 in]
    n13 = call-poly <vilib>:"Write To Spreadsheet File.vi"("format (%.3f)"="%.5f", "2D data"=w18) -> ()  [unwired: 6 in, 1 out]
  }
  n14 = call "Convert to Dynamic Data2"("2D Array"=w2) -> ("Dynamic Data Type"=w16:dynamicdata)  [unwired: 3 in]
  n15 = call "Convert to Dynamic Data"("2D Array"=w3) -> ("Dynamic Data Type"=w17:dynamicdata)  [unwired: 3 in]
  n16 = call "Build XY Graph"("Y Input"=w16, "X Input"=w17) -> ("XY Graph"=→"XY Graph":cluster{"Y":dbl[], "Y":dbl[]}[])  [unwired: 8 in, 1 out]
